vi "CaLabDisconnect_PV-1D.vi"(10 "All PVs? (No)":bool, 11 "PV Names":string[](array[string])) -> ()   [LabVIEW 2022 SP3, in "CaLab.lvlib"]
doc: "This is a VI for disconnecting EPICS variables.\n\n<b>INPUT:</b>\n <b>PV Name(s)</b>\n String array of EPICS variable names\n <b>all (false)</b>\n TRUE: Disconnect all EPICS variables"
uses:
  CaLab.lvlib
  <userlib>/calab/lib/calab.dll
panel:
  out "error out":errorcluster
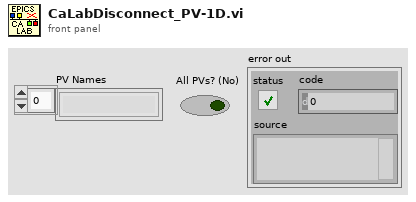
[diagram p1: front panel]
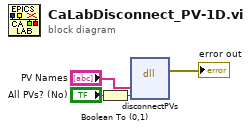
[diagram p0: block diagram]
diagram:
  n1 = Boolean To (0,1)(Boolean="All PVs? (No)") -> (0, 1=w2:i16)
  n2 = dll-call lib="C:/Program Files/National Instruments/LabVIEW 2023/user.lib/calab/lib/calab.dll" fn="disconnectPVs" label="caLabDisconnect"("PVNameArray"="PV Names", "All"=w2) -> (error out=→"error out":errorcluster)  [unwired: 5 in, 2 out]
